vi "Standard Event Register Query.vi"(0 "VISA resource name":refnum<visa-resource-name>="COM1", 11 "error in (no error)":errorcluster) -> (4 "VISA resource name out":refnum<visa-resource-name>="COM1", 6 "Standard Event Register":T1, 15 "error out":errorcluster)   [LabVIEW 2014, in "Associated Power Technologies 8500 Series.lvlib"]
doc: "Queries the Event Status Register and returns the byte data available in it.\nEach bit represent the occurrence of an event.\n\nEx : BIT 0 is set High when \"Operation Complete\"\n\nBIT 0 ,01H, (1) Operation Complete\nBIT 1 ,02H, (2) Not Used\nBIT 2 ,04H, (4) Query Error\nBIT 3 ,08H, (8) Device Error\nBIT 4 ,10H,(16) Execution Error\nBIT 5 ,20H,(32) Command Error\nBIT 6 ,40H,(64) Not Used\nBIT 7 ,80H,(128) Power On"
uses:
  <instrlib>/Associated Power Technologies 8500 Series/Associated Power Technologies 8500 Series.lvlib
panel:
  # "BIT 0 ,01H, (1)    Operation Complete\nBIT 1 ,02H, (2)    Not Used\nBIT 2 ,04H, (4)    Query Error\nBIT 3 ,08H, (8)    Device Error\nBIT 4 ,10H,(16)   Execution Error\nBIT 5 ,20H,(32)   Command Error\nBIT 6 ,40H,(64)   Not Used\nBIT 7 ,80H,(128)  Power On"
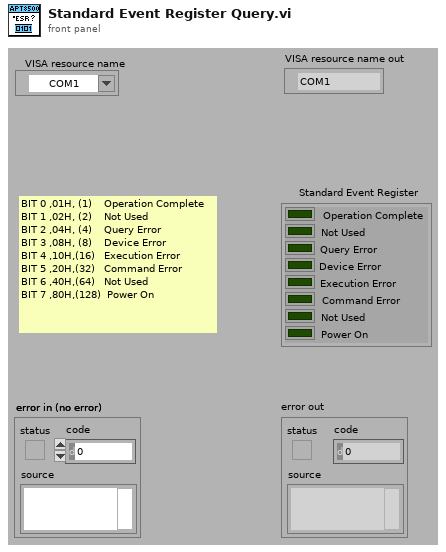
[diagram p1: front panel]
types:
  T1 = cluster{"Operation Complete":bool, "Not Used":bool, "Query Error":bool, "Device Error":bool, "Execution Error":bool, "Command Error":bool, "Not Used":bool, "Power On":bool}
  T2 = cluster{"Boolean array[0]":bool, "Boolean array[1]":bool, "Boolean array[2]":bool, "Boolean array[3]":bool, "Boolean array[4]":bool, "Boolean array[5]":bool, "Boolean array[6]":bool, "Boolean array[7]":bool}
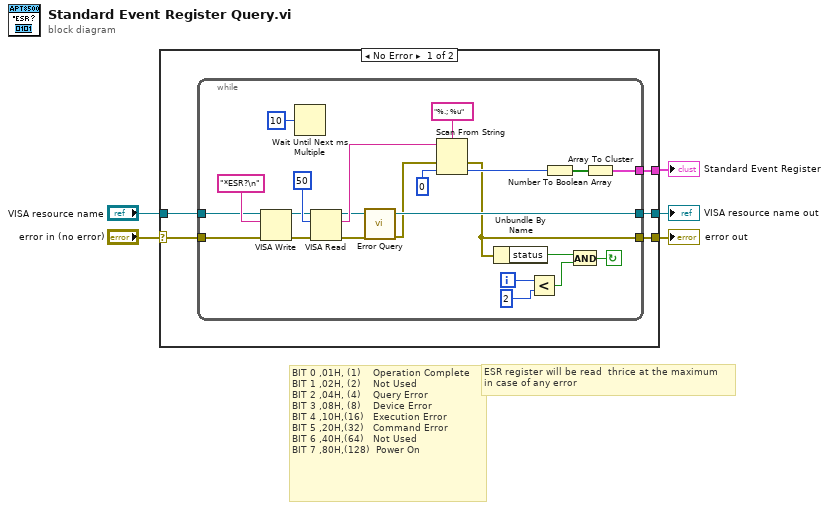
[diagram p0: block diagram]
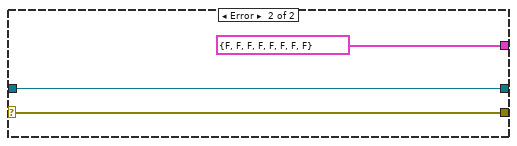
[diagram p2: hidden frame]
diagram:
  # "ESR register will be read  thrice at the maximum\nin case of any error"
  # "BIT 0 ,01H, (1)    Operation Complete\nBIT 1 ,02H, (2)    Not Used\nBIT 2 ,04H, (4)    Query Error\nBIT 3 ,08H, (8)    Device Error\nBIT 4 ,10H,(16)   Execution Error\nBIT 5 ,20H,(32)   Command Error\nBIT 6 ,40H,(64)   Not Used\nBIT 7 ,80H,(128)  Power On"
  n1 = case shown="No Error" "error in (no error)" {
    selector: "error in (no error)" -> [w7 w36]
    tunnel: [w10 T2 {"Boolean array[0]"=FALSE, "Boolean array[1]"=FALSE, "Boolean array[2]"=FALSE, "Boolean array[3]"=FALSE, "Boolean array[4]"=FALSE, "Boolean array[5]"=FALSE, "Boolean array[6]"=FALSE, "Boolean array[7]"=FALSE} ("Boolean array")] -> w1
    tunnel: [w8 w36] -> w2
    tunnel: "VISA resource name" -> [w6 w35]
    tunnel: [w9 w35] -> w4
    frame No Error {
      n2 = while {
        tunnel: [w30] -> w10
        tunnel: w6 -> [w18]
        tunnel: [w15] -> w9
        tunnel: w7 -> [w20]
        tunnel: [w11] -> w8
        i -> [w26]
        stop <- w22 continue-if-true
        n3 = VISA Write(VISA resource name=w18, write buffer="*ESR?\n" ("Command to Send (empty)"), error in (no error)=w20) -> (VISA resource name out=w17:refnum<visa-resource-name>, error out=w19:errorcluster)  [unwired: 1 out]
        n4 = Wait Until Next ms Multiple(millisecond multiple=u32 10) -> ()  [unwired: 1 out]
        n5 = VISA Read(VISA resource name=w17, byte count=u32 50, error in (no error)=w19) -> (VISA resource name out=w13:refnum<visa-resource-name>, read buffer=w32:string, error out=w14:errorcluster)  [unwired: 1 out]
        n6 = call <instrlib>:"Error Query.vi"("VISA resource name"=w13, "error in (no error)"=w14) -> ("VISA resource name out"=w15:refnum<visa-resource-name>, "error out"=w12:errorcluster)  [unwired: 10 in, 2 out]
        n7 = Scan From String(format string="%.; %u" ("Format String"), input string=w32, error in=w12, default 1=u8 0 ("default value 1")) -> (error out=w11:errorcluster, output 1=w27:u8)  [unwired: 1 in, 2 out]
        n8 = Unbundle By Name(w11) -> ("status"=w23:bool)
        n9 = Less?(x=w26, y=2) -> (x < y?=w24:bool)
        n10 = Number To Boolean Array(number=w27) -> (Boolean array=w31:bool[])
        n11 = And(x=w23, y=w24) -> (x .and. y?=w22:bool)
        n12 = Array To Cluster(array=w31) -> (cluster=w30:T2)
      }
    }
    frame Error {
    }
  }
  "Standard Event Register" <- w1
  "VISA resource name out" <- w4
  "error out" <- w2
